vi "App_Ref_Global.vi"(2 "Input Array":T1[](array[typedef]), 3 "Mode":T2) -> (0 "Output Array":T1[](array[typedef]))   [LabVIEW 2010]
uses:
  Controls/App_Global.ctl
  Controls/App_Ref_Cluster.ctl
  Controls/Serveds.ctl
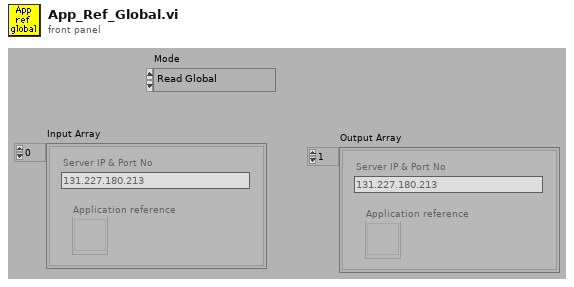
[diagram p1: front panel]
types:
  T1 = typedef "App_Ref_Cluster.ctl" = cluster{"Server IP & Port No":string, "Application reference":refnum<vi>}
  T2 = typedef "App_Global.ctl" = enum16{"Read Global", "Write to Global", "Initialise Array"}
  T3 = typedef "Serveds.ctl" = enum16{"Read Global", "Load Global From File"}
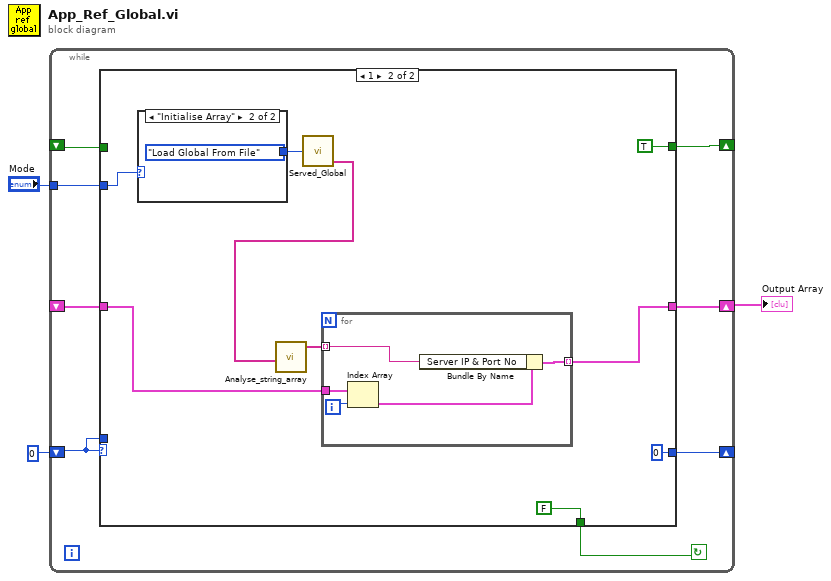
[diagram p0: block diagram]
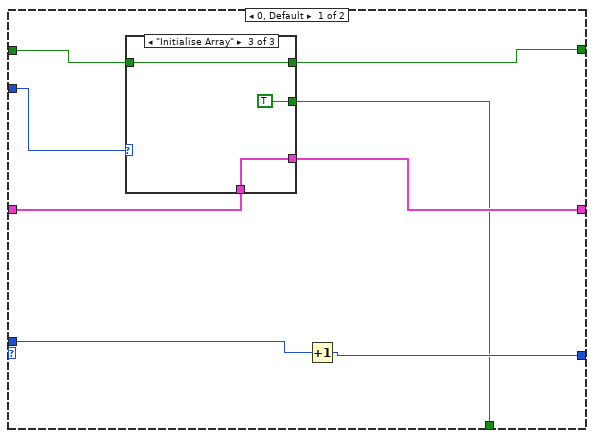
[diagram p2: hidden frame]
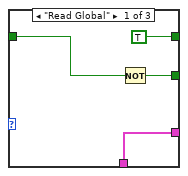
[diagram p3: hidden frame]
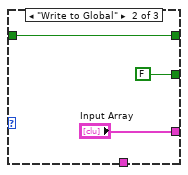
[diagram p4: hidden frame]
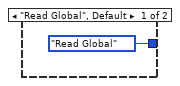
[diagram p5: hidden frame]
diagram:
  n1 = while {
    tunnel: "Mode" -> [w5]
    shift-left: 0 -> [w6]
    shift-right: [w8] -> _
    shift-left: _ -> [w10]
    shift-right: [w7] -> w1
    shift-left: _ -> [w11]
    shift-right: [w4] -> _
    stop <- w9 continue-if-true
    n2 = case shown="1" w6 {
      tunnel: w11 -> [w13 _]
      tunnel: w10 -> [w15 w31]
      tunnel: [w14 FALSE] -> w9
      tunnel: [w18 0] -> w8
      tunnel: [w16 w30] -> w7
      tunnel: w6 -> [w19 _]
      tunnel: w5 -> [w17 w34]
      tunnel: [w12 TRUE] -> w4
      frame 0, Default {
        n3 = case shown="\"Initialise Array\"" w17 {
          tunnel: [w23 "Input Array" w27] -> w16
          tunnel: w15 -> [w23 _ w27]
          tunnel: [w21 FALSE TRUE] -> w14
          tunnel: w13 -> [w22 w24 w29]
          tunnel: [TRUE w24 w29] -> w12
          frame "Read Global" {
            n4 = Not(x=w22) -> (.not. x?=w21:bool)
          }
          frame "Write to Global" {
          }
          frame "Initialise Array" {
          }
        }
        n5 = Increment(x=w19) -> (x+1=w18:i32)
      }
      frame 1 {
        n6 = case shown="\"Initialise Array\"" w34 {
          tunnel: [Serveds."Read Global" ("Mode") Serveds."Load Global From File" ("Mode")] -> w33
          frame "Read Global", Default {
          }
          frame "Initialise Array" {
          }
        }
        n7 = call "Served_Global.vi"("Mode"=w33) -> ("Served IP Number & Port No"=w32:string[])  [unwired: 2 out]
        n8 = call "Analyse_string_array.vi"("String array"=w32) -> ("Unique strings"=w37:string[])  [unwired: 2 out]
        n9 = for {
          tunnel: w37 -> [w42] mode=indexing
          tunnel: w31 -> [w44]
          tunnel: [w41] -> w30 mode=indexing
          i -> [w45]
          n10 = Index Array(array=w44, index=w45) -> (element=w43:T1)
          n11 = Bundle By Name(cluster=w43, "Server IP & Port No"=w42) -> (w41:T1)
        }
      }
    }
  }
  "Output Array" <- w1
